vi "Pre Launch Init.vi"(11 "Simple Chat in":refnum<class "Simple Chat.lvclass">) -> (0 "error out":errorcluster, 3 "Simple Chat out":refnum<class "Simple Chat.lvclass">)   [LabVIEW 2020, in "Simple Chat.lvlib" / "Simple Chat.lvclass"]
doc: "(<B>Filename</B>: Actor Framework.lvlib:Actor.lvclass:Pre Launch Init.vi)\n\nDefines behavior that occurs after the Launch Nested Actor method is invoked but before the actor's Actor Core method begins running.\n\nBy default, this method does nothing. A descendant class may override it to define behavior."
uses:
  Simple Chat.lvclass
  C:/Program Files/National Instruments/LabVIEW 2020/vi.lib/ActorFramework/Actor/Actor.lvclass
  <vilib>/ActorFramework/Stop Msg/Stop Msg.lvclass
  C:/Program Files/National Instruments/LabVIEW 2020/vi.lib/ActorFramework/Message/Message.lvclass
  Actor Pub Sub Channels/Pub Sub Retaining Message Channel/Pub Sub Retaining Message Channel.lvclass
  E:/Labview/LV 2020/Libs/Actor Pub Sub/Source/Actor Pub Sub Channels/Pub Sub Message Channel/Pub Sub Message Channel.lvclass
  Message Reciever Interface/Message Reciever Interface.lvclass
  <vilib>/ActorFramework/Actor/Actor.lvclass/Actor.ctl
  <vilib>/ActorFramework/Message Enqueuer/Message Enqueuer.lvclass/Message Enqueuer.ctl
  Simple Chat.lvclass/Simple Chat.ctl
  848bf2ce-151b-44f6-88e3-c0d6abaf681b.vi
  bbcedd2a-a366-49d9-a7cd-f1a423d06d3f.vi
  <vilib>/ActorFramework/Message Enqueuer/Init from Existing Queue.vi
  bbcedd2a-a366-49d9-a7cd-f1a423d06d3f.vi/ab9dd782-548d-4861-b01d-d668ac712bc7.vi
  Actor Pub Sub Channels/Helpers/Subscribe Actor to Class Topic.vi
  Actor Pub Sub Channels/Helpers/Subscribe Actor to Topic.vi
  <vilib>/ActorFramework/Actor/Actor.lvclass
  <vilib>/ActorFramework/Message Enqueuer/Message Enqueuer.lvclass
  <vilib>/ActorFramework/Message/Message.lvclass
  Actor Pub Sub Channels/Actor Pub Sub Channels.lvlib
  Actor Pub Sub Channels/Pub Sub Message Channel/Pub Sub Message Channel.lvclass
  E:/Labview/LV 2020/Libs/Actor Pub Sub/Source/Actor Pub Sub Channels/Pub Sub Retaining Message Channel/Pub Sub Retaining Message Channel.lvclass
  C:/Program Files/National Instruments/LabVIEW 2020/vi.lib/ActorFramework/Stop Msg/Stop Msg.lvclass
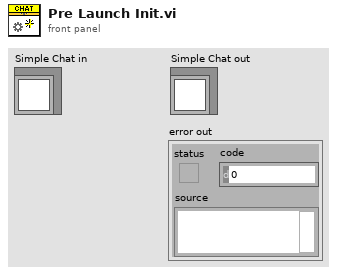
[diagram p1: front panel]
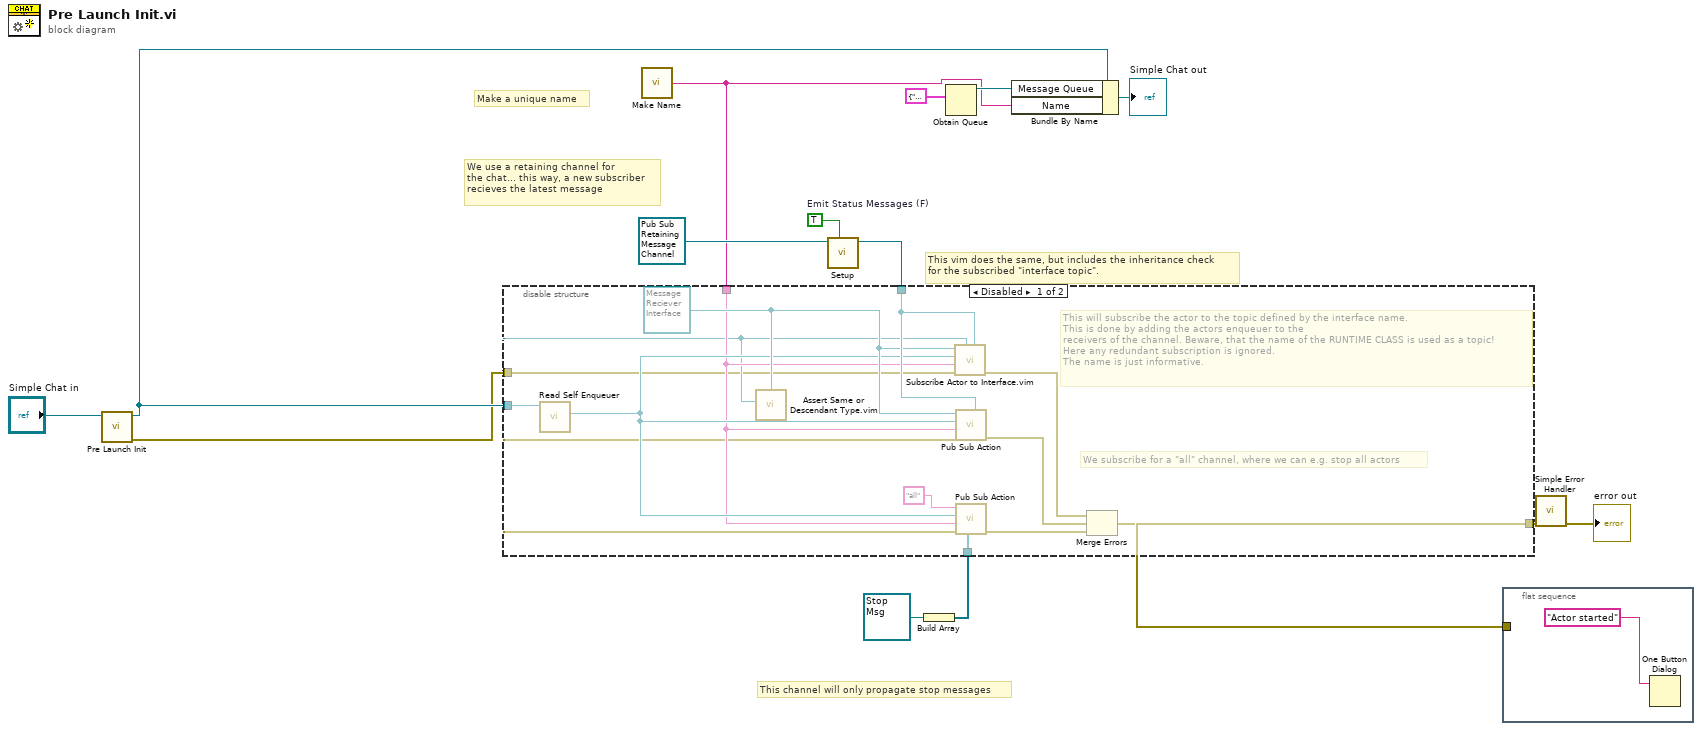
[diagram p0: block diagram]
diagram:
  w9 = TRUE  # Emit Status Messages (F)
  # "This channel will only propagate stop messages"
  # "Make a unique name"
  # "We use a retaining channel for\nthe chat... this way, a new subscriber\nrecieves the latest message"
  # "This vim does the same, but includes the inheritance check\nfor the subscribed \"interface topic\"."
  n1 = call-parent "Pre Launch Init.vi"("Actor in"="Simple Chat in") -> ("error out"=w3:errorcluster, "Actor out"=w6:refnum<class "Simple Chat.lvclass">)  [unwired: 9 in]
  n2 = call "Make Name.vi"() -> ("Actor Name"=w7:string)
  n3 = call "Setup.vi"("Emit Status Messages (F)"=w9, "Pub Sub Message Channel in"=refnum<class "Pub Sub Retaining Message Channel.lvclass"> refnum ("Actor Pub Sub Channels.lvlib:Pub Sub Retaining Message Channel.lvclass")) -> ("Pub Sub Message Channel out"=w10:refnum<class "Pub Sub Retaining Message Channel.lvclass">)  [unwired: 8 in, 1 out]
  n4 = Build Array(refnum<class "Stop Msg.lvclass"> refnum ("Actor Framework:Stop Msg")) -> (w4:refnum<class "Stop Msg.lvclass">[])
  n5 = disable-structure shown="Disabled" {
    disable-tunnel: w10 -> [w26 _]
    disable-tunnel: w7 -> [w22 _]
    disable-tunnel: w6 -> [w21 _]
    disable-tunnel: w4 -> [w20 _]
    disable-tunnel: w3 -> [w19 _]
    disable-tunnel: [w15 _] -> w1
    frame Disabled {
      w25 = refnum<class "Message Reciever Interface.lvclass"> refnum ("Simple Chat.lvlib:Message Reciever Interface.lvclass")
      # "We subscribe for a \"all\" channel, where we can e.g. stop all actors"
      # "This will subscribe the actor to the topic defined by the interface name.\nThis is done by adding the actors enqueuer to the\nreceivers of the channel. Beware, that the name of the RUNTIME CLASS is used as a topic!\nHere any redundant subscription is ignored.\nThe name is just informative."
      n6 = call <vilib>:"Read Self Enqueuer.vi"("Actor"=w21) -> ("Self Enqueuer"=w23:refnum<class "Message Enqueuer.lvclass">)  [unwired: 10 in]
      n7 = call "Assert Same or Descendant Type.vim"("ancestor type"=w25, "value in"=w21) -> ()  [unwired: 7 in, 1 out]
      n8 = call "Subscribe Actor to Interface.vim"("Channel Class"=w26, "Actor"=w21, "error in (no error)"=w19, "Name"=w22, "Receivers Enqueuer"=w23, "Topic"=w25) -> ("error out"=w17:errorcluster)  [unwired: 4 in, 1 out]
      n9 = call-poly "Pub Sub Action.vi"("Channel Class"=w26, "error in (no error)"=w19, "Name"=w22, "Receivers Enqueuer"=w23, "Topic"=w25) -> ("error out"=w16:errorcluster)  [unwired: 5 in, 1 out]
      n10 = call-poly "Pub Sub Action.vi"("Included (All)"=w20, "error in (no error)"=w19, "Name"=w22, "Receivers Enqueuer"=w23, "Topic"="all") -> ("error out"=w18:errorcluster)  [unwired: 4 in, 2 out]
      n11 = Merge Errors(w17, w16, w18) -> (w15:errorcluster)
    }
    frame Enabled {
    }
  }
  n12 = Obtain Queue(element data type=cluster{"Sender":string, "Message":string} {"Sender"="", "Message"=""}) -> (queue out=w11:refnum<queue>)  [unwired: 4 in, 2 out]
  n13 = Bundle By Name(cluster=w6, "Message Queue"=w11, "Name"=w7) -> (→"Simple Chat out":refnum<class "Simple Chat.lvclass">)
  n14 = flat-sequence {
    tunnel: w1 -> [_]
    frame #0 {
      n15 = One Button Dialog(message="Actor started") -> ()  [unwired: 1 in, 1 out]
    }
  }
  n16 = call <vilib>:"Simple Error Handler.vi"("error in (no error)"=w1) -> ("error out"=→"error out":errorcluster)  [unwired: 4 in, 4 out]
